vi "CryoCooler_AVC_Serial_Write_and_Read.vi"(8 "error in (no error)":errorcluster, 9 "Command Options":string, 10 "Command":T1 items=["STATUS", "COOLER", "E", "ERROR", "KD", "KI", "KP", "LOGIN", "LOGOUT", "MODE", "P", "PWOUT", "SENSOR", "TC", "TEMP RJ", "TTARGET", "VERSION"], 11 "VISA Resource (write)":refnum<visa-resource-name>="COM1") -> (0 "error out":errorcluster, 2 "VISA Resource out":refnum<visa-resource-name>="COM1", 3 "read string array":string[](array[string]))   [LabVIEW 2020]
doc: "This example opens two VISA resources and configures one COM port to perform a write operation and the other COM port to perform a read operation. This VI will wait until the specified number of bytes is received at the port or until a termination character is read.\n\nThis example allows you perform diagnostic tests on your ports. You can use this example to perform a wrap-back test. Both serial ports must have the same basic configuration parameters. You can connect two of the ports using a null modem cable, which effectively connects one port's RX lines to the other port's TX lines. If you use a straight-through cable, one port's RX lines will be connected to the other port's RX lines, and you cannot communicate between the two ports."
uses:
  Cryo Cooler/CryoCoolerAVC/CryoCoolerAVC Command enum.ctl
  VIs/PRIME/PRIME/Cryotel/Cooler_control/Serial - Settings.ctl
  <vilib>/Instr/_visa.llb/VISA Configure Serial Port (Instr).vi
panel:
  in  "Custom Command":string
  out "bytes read array":u32[](array[numeric])
  out "Read String":string
  in  "End Write on Termination Character?":bool=TRUE
  in  "End Read on Termination Character?":bool=TRUE
  out "bytes read":u32
  out "bytes written":u32
  in  "Tab Control":enum32{"Standard command", "Custom command"}(tab)
  in  "Lines to read":u16
  # "Overview: Demonstrates the use of the VISA functions to communicate between two different serial devices.\nRequirements: NI-VISA Driver, two serial devices\nInstructions:\n1. Ensure the resources specified by VISA Resource (write) and VISA Resource (read) are valid serial devices.\n2. Connect a null modem RS-232 or RS-485/422 cable between the 2 ports.\n3. Run the VI.\n4. If your two devices are connected properly, you should see the Read String value match the Write String value."
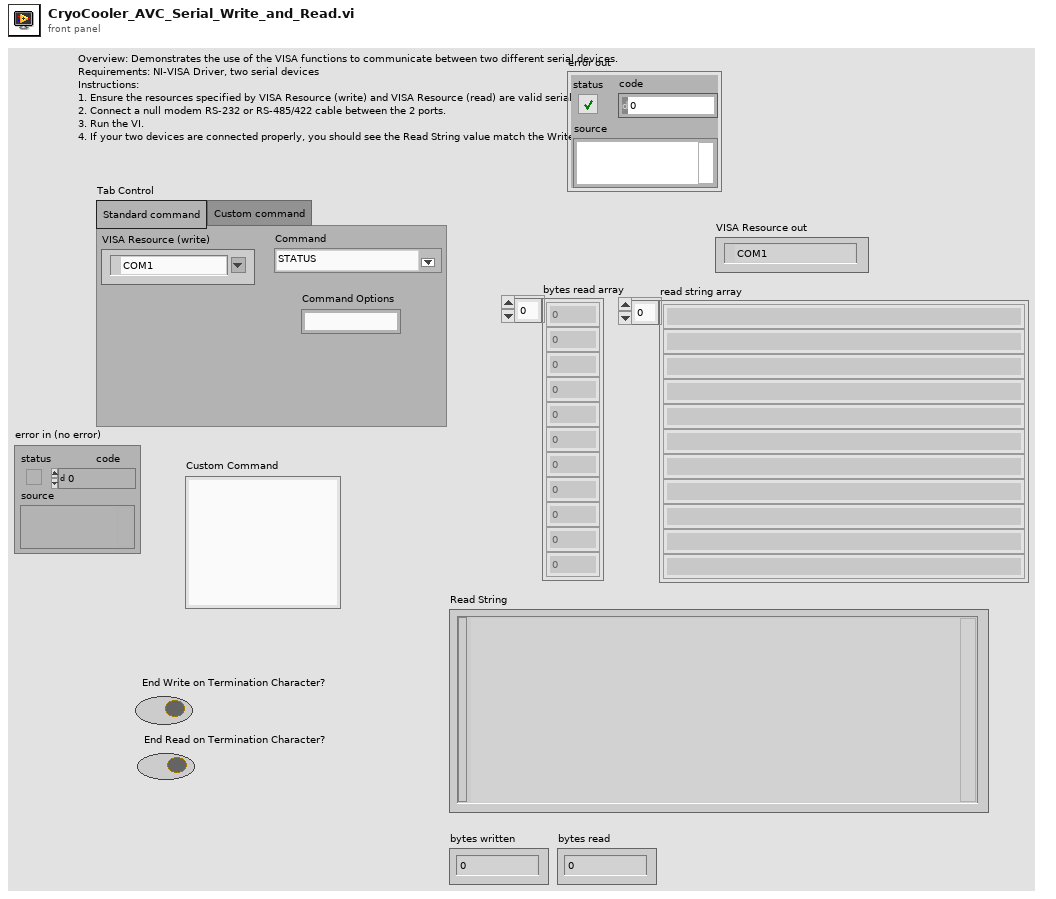
[diagram p1: front panel]
types:
  T1 = typedef "CryoCoolerAVC Command enum.ctl" = u16
  T2 = typedef "Serial - Settings.ctl" = cluster{"baud rate":u32, "data bits":u16, "parity":enum16{"None", "Odd", "Even", "Mark", "Space"}, "stop bits":u16, "flow control":u16}
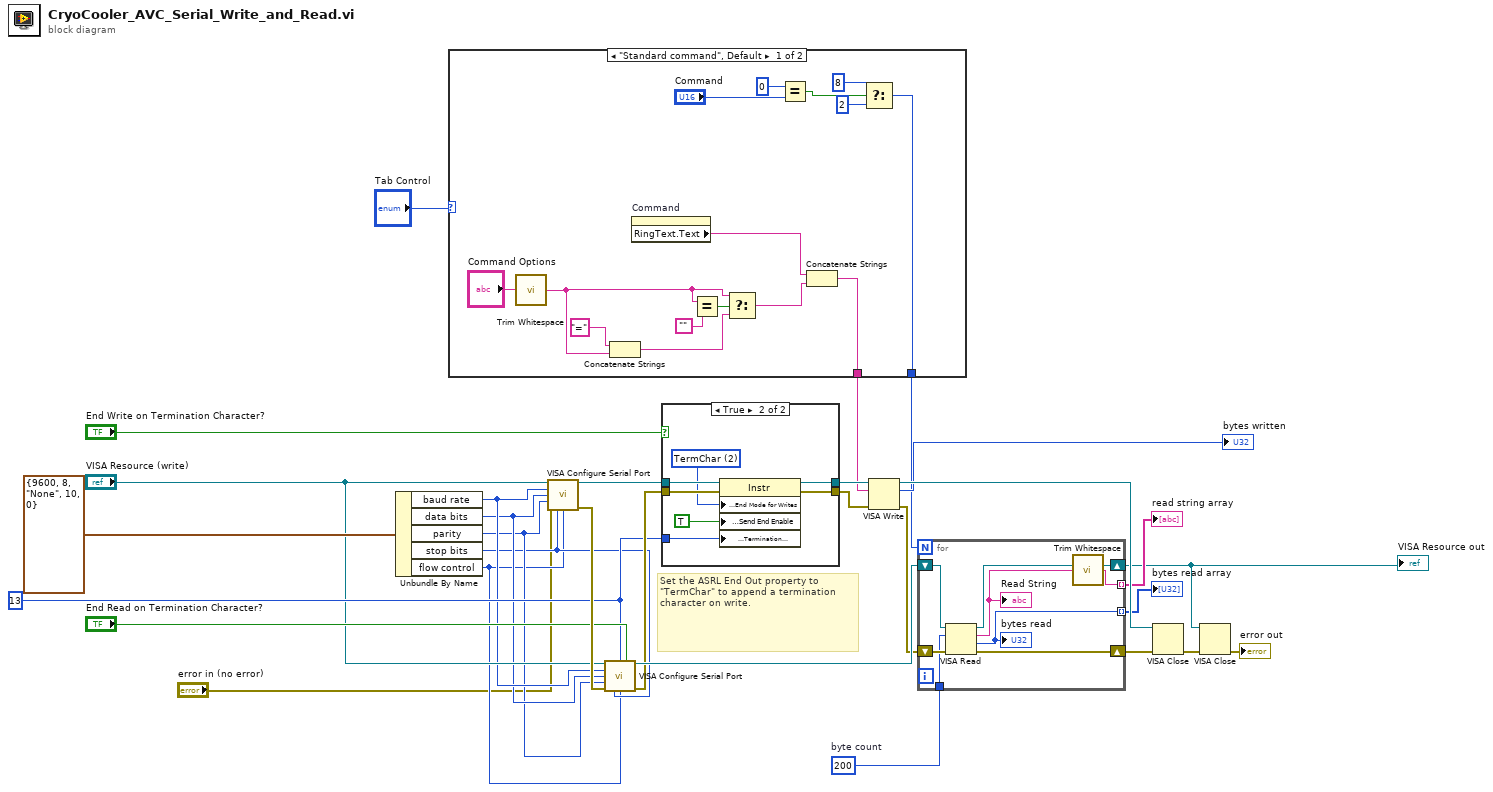
[diagram p0: block diagram]
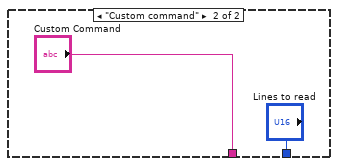
[diagram p2: hidden frame]
diagram:
  w16 = u8 13 ("Termination Character")
  w7 = u32 200  # byte count
  # "Set the ASRL End Out property to \"TermChar\" to append a termination character on write."
  n1 = Unbundle By Name(T2 {"baud rate"=9600, "data bits"=8, "parity"=enum."None", "stop bits"=10, "flow control"=0} ("Serial Settings (write)")) -> ("baud rate"=w14:u32, "data bits"=w13:u16, "parity"=w12:enum16{"None", "Odd", "Even", "Mark", "Space"}, "stop bits"=w11:u16, "flow control"=w10:u16)
  n2 = case shown="\"Standard command\", Default" "Tab Control" {
    tunnel: [w40 "Lines to read"] -> w6
    tunnel: [w31 "Custom Command"] -> w5
    frame "Standard command", Default {
      n3 = call <vilib>:"Trim Whitespace.vi"("string"="Command Options") -> ("trimmed string"=w35:string)  [unwired: 1 in]
      n4 = Concatenate Strings("=" ("string"), w35) -> (w36:string)
      n5 = property on="Command" class="Ring (strict)"() -> ("RingText.Text"=w32:string)  [unwired: 2 in, 2 out]
      n6 = Equal?(x=w35, y="") -> (x = y?=w37:bool)
      n7 = Select(t=w35, s=w37, f=w36) -> (s? t:f=w33:string)
      n8 = Equal?(x=u16 0, y="Command") -> (x = y?=w43:bool)
      n9 = Concatenate Strings(w32, w33) -> (w31:string)
      n10 = Select(t=u16 8 ("x"), s=w43, f=u16 2) -> (s? t:f=w40:u16)
    }
    frame "Custom command" {
    }
  }
  n11 = call-poly "VISA Configure Serial Port"("VISA resource name"="VISA Resource (write)", "baud rate (9600)"=w14, "data bits (8)"=w13, "parity (0:none)"=w12, "error in (no error)"="error in (no error)", "stop bits (10: 1 bit)"=w11, "flow control (0:none)"=w10) -> ("VISA resource name out"=w21:refnum<visa-resource-name>, "error out"=w27:errorcluster)  [unwired: 2 in, 5 out]
  n12 = call-poly "VISA Configure Serial Port"("VISA resource name"="VISA Resource (write)", "termination char\n(0xA = '\\n' = LF)"=w16, "Enable Termination\nChar (T)"="End Read on Termination Character?", "baud rate (9600)"=w14, "data bits (8)"=w13, "parity (0:none)"=w12, "error in (no error)"=w27, "stop bits (10: 1 bit)"=w11, "flow control (0:none)"=w10) -> ("VISA resource name out"=w29:refnum<visa-resource-name>, "error out"=w19:errorcluster)  [unwired: 1 in, 4 out]
  n13 = case shown="True" "End Write on Termination Character?" {
    tunnel: w21 -> [w48 w56]
    tunnel: w19 -> [w49 w55]
    tunnel: [w48 w54] -> w20
    tunnel: [w49 w53] -> w18
    tunnel: w16 -> [_ w51]
    frame False {
    }
    frame True {
      w52 = u16 2 items=["None", "LastBit", "TermChar", "Break"] ("Serial Settings:Serial End Mode for Writes")
      n14 = property class="Instr"(reference=w56, error in=w55, "Serial Settings:End Mode for Writes"=w52, "Message Based Settings:Send End Enable"=TRUE, "Message Based Settings:Termination Character"=w51) -> (reference out=w54:refnum<visa-resource-name>, error out=w53:errorcluster)
    }
  }
  n15 = VISA Write(VISA resource name=w20, write buffer=w5, error in (no error)=w18) -> (VISA resource name out=w30:refnum<visa-resource-name>, return count=→"bytes written":u32, error out=w26:errorcluster)
  n16 = for {
    N: w6 -> [_]
    tunnel: [w57] -> w9 mode=indexing
    shift-right: [w63] -> w3
    shift-left: w29 -> [w64]
    shift-right: [w61] -> w25
    shift-left: w26 -> [w62]
    tunnel: [w59] -> w8 mode=indexing
    tunnel: w7 -> [w58]
    n17 = VISA Read(VISA resource name=w64, byte count=w58, error in (no error)=w62) -> (VISA resource name out=w63:refnum<visa-resource-name>, read buffer=w60:string, return count=w59:u32, error out=w61:errorcluster)
    "Read String" <- w60
    "bytes read" <- w59
    n18 = call <vilib>:"Trim Whitespace.vi"("string"=w60) -> ("trimmed string"=w57:string)  [unwired: 1 in]
  }
  "read string array" <- w9
  "bytes read array" <- w8
  "VISA Resource out" <- w3
  n19 = VISA Close(VISA resource name=w30, error in (no error)=w25) -> (error out=w24:errorcluster)
  n20 = VISA Close(VISA resource name=w3, error in (no error)=w24) -> (error out=→"error out":errorcluster)
